vi "Accelerator Complex Process.vi"(9 "Sessions Parameters":T1={"intra_op_num_threads"=0, "inter_op_num_threads"=0, "execution_mode"=enum."ORT_SEQUENTIAL", "deterministic_compute"=FALSE, "graph_optimization_level"=1, "optimized_model_file_path"=path "", "profiling output dir"=path ""} {"graph_optimization_level" items=["ORT_DISABLE_ALL"=0, "ORT_ENABLE_ALL"=1, "ORT_ENABLE_BASIC"=2, "ORT_ENABLE_EXTENDED"=99]}, 10 "Execution Device":enum16{"CPU", "NVIDIA CUDA", "NVIDIA TensorRT"}(ring)=enum."NVIDIA CUDA", 11 "X size":i32=16384) -> (3 "Accelerator Time":dbl=1.5238084999999728)   [LabVIEW 2020]
uses:
  <vilib>/Graiphic/Accelerator/Source/ONNX/_Controls/acc_CUDA_ep_params_simplified.ctl
  <vilib>/Graiphic/Accelerator/Source/ONNX/_Controls/acc_tensorRT_ep_params_simplified.ctl
  <vilib>/Graiphic/Accelerator/Source/SubVIs/add_to_cluster_onnx_input/acc_onnx_add_1d_complexfloat_array_into_ptr_input_cluster_array_by_idx.vi
  <vilib>/Graiphic/Accelerator/Source/Model/_Methods/acc_create_onnx_model_then_init_cuda_inference_session.vi
  <vilib>/Graiphic/Accelerator/Source/Model/_Methods/acc_create_onnx_model_then_init_cpu_inference_session.vi
  <vilib>/Graiphic/Accelerator/Source/Model/_Methods/acc_create_onnx_model_then_init_tensorRT_inference_session.vi
  <vilib>/Graiphic/Accelerator/Source/SubVIs/add_to_cluster_onnx_input/acc_onnx_add_scalar_complexfloat_array_into_ptr_input_cluster_array_by_idx.vi
  <vilib>/Graiphic/Accelerator/Source/ONNX/Inference/_Methods/Simplified/acc_embedded_run_preallocated_multi_input_and_outputs_gpu_by_idx.vi
  <vilib>/Graiphic/Accelerator/Source/ONNX/Inference/_Methods/Exec_GPU/acc_embedded_copy_cuda_ptr_data_to_labview_data.vi
  <vilib>/Graiphic/Accelerator/Source/ONNX/Inference/_Methods/Simplified/acc_embedded_run_mono_output_scalar_complexfloat.vi
  <vilib>/Graiphic/Accelerator/Source/ONNX/Inference/acc_Inference.lvclass
  <vilib>/Graiphic/Accelerator/Source/Model/acc_Model.lvclass
  <vilib>/Analysis/NI_AALBase.lvlib
panel:
  in  "nb_loop":i32=6
  out "max value":csg=1.3257894e+20+1.4545643e+21i
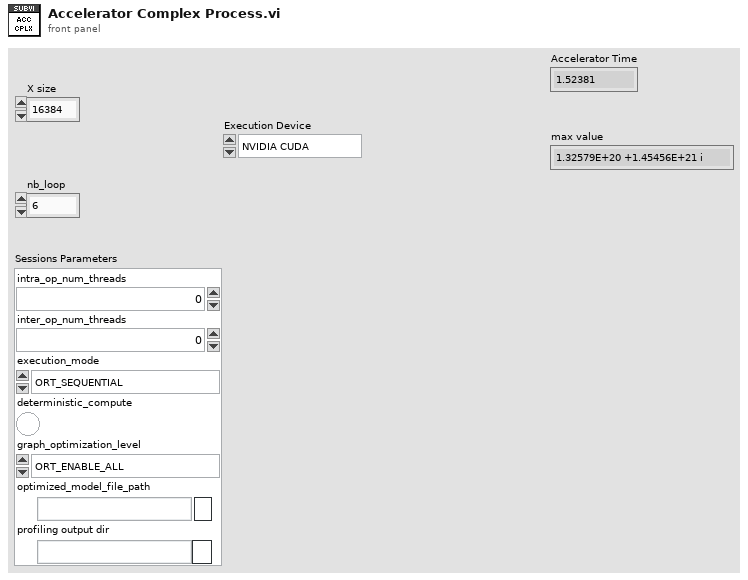
[diagram p1: front panel]
types:
  T1 = cluster{"intra_op_num_threads":i32, "inter_op_num_threads":i32, "execution_mode":enum16{"ORT_SEQUENTIAL", "ORT_PARALLEL"}, "deterministic_compute":bool, "graph_optimization_level":u16, "optimized_model_file_path":path, "profiling output dir":path}
  T2 = typedef "acc_onnx_multi_ptr_input_index_cluster.ctl" = cluster{"input_order":u32, "Inputs Info":cluster{"inputs_ptr":u64, "inputs_shapes":i64[], "inputs_ranks":i64, "inputs_types":T3}}
  T3 = typedef "acc_onnx_dtype_enum.ctl" = enum16{"UNDEFINED", "FLOAT", "UINT8", "INT8", "UINT16", "INT16", "INT32", "INT64", "STRING", "BOOL", "FLOAT16", "DOUBLE", "UINT32", "UINT64", "COMPLEX64", "COMPLEX128", "BFLOAT16", "FLOAT8E4M3FN", "FLOAT8E4M3FNUZ", "FLOAT8E5M2", "FLOAT8E5M2FNUZ", "UINT4", "INT4"}
  T4 = typedef "acc_CUDA_ep_params_simplified.ctl" = cluster{"Device & Stream":cluster{"Device Index":i32, "Use Custom Compute Stream?":bool, "Custom Compute Stream (Pointer)":u64, "Copy Using Default Stream?":bool}, "Memory Management":cluster{"GPU Memory Limit (Bytes)":u64, "Arena Extension Strategy":enum16{"kNextPowerOfTwo", "kSameAsRequested"}, "Default Memory Arena Config":u64}, "CuDNN & Kernel Optimization":cluster{"cuDNN Convolution Algorithm Search":enum16{"OrtCudnnConvAlgoSearchExhaustive", "OrtCudnnConvAlgoSearchHeuristic", "OrtCudnnConvAlgoSearchDefault"}, "Use Max Workspace for cuDNN?":bool, "Pad Conv1D Inputs to NC1D?":bool, "Fuse Convolution + Bias?":bool, "Scaled Dot-Product Attention Kernel Option":bool, "Enable Strict SkipLayerNorm Mode?":bool}, "Execution & Precision Controls":cluster{"Enable CUDA Graph Execution?":bool, "Use EP-Level Unified Stream?":bool, "Prefer NHWC Tensor Layout?":bool, "Use TensorFloat-32 (TF32)?":bool}, "Tunable Operator System":cluster{"Enable Tunable Operators?":bool, "Enable Tuning Mode for Tunable Operators?":bool, "Max Tuning Duration (ms)":i32}}
  T5 = typedef "acc_tensorRT_ep_params_simplified.ctl" = cluster{"Device And Stream":cluster{"Device Index":i32, "Use Custom Compute Stream?":bool, "Custom Compute Stream (Pointer)":u64}, "Parser & Subgraph Options":cluster{"Max Partition Attemps":i32, "Minimum Subgraph Size":i32}, "Memory & Workspace Management":cluster{"Max Workspace Memory (Bytes)":u64, "Share Memory Between Subgraphs":bool, "Auxiliary Stream Count":i32}, "Precision & Numeric Modes":cluster{"Enable FP16":bool, "Enable BF16":bool, "Enable INT8":bool, "INT8 Calibration Table Name":path, "Use Native INT8 Calibration?":bool}, "Engine Build, Cache & Paths":cluster{"Enable Engine Caching?":bool, "Engine Cache Directory":path, "Enable Engine Decryption?":bool, "Decryption Library Path":path, "Build Engines Sequentially?":bool, "Enable Timing Cache?":bool, "Timing Cache Directory":path, "Force Timing Cache Use?":bool, "Enable Detailed Logs?":bool, "Use Build Heuristics?":bool, "Enable Weight Sparsity?":bool, "Engine Optimization Level (0–5)":i32}, "Paths & Plugins":cluster{"Extra Plugin Libraries":path[], "Tactic Source Rules":string, "Enabled Preview Features":enum16{"None", "ALIASED_PLUGIN_IO_10_03"}}, "Profile Shapes":cluster{"Minimum Input Shapes":string, "Maximum Input Shapes":string, "Optimal Input Shapes":string}, "Advanced & DLA / CUDA Graph":cluster{"Enable DLA Acceleration?":bool, "DLA Core Index":i32, "Dump TensorRT Subgraphs?":bool, "Force LayerNorm in FP32?":bool, "Enable CUDA Graph Execution?":bool}}
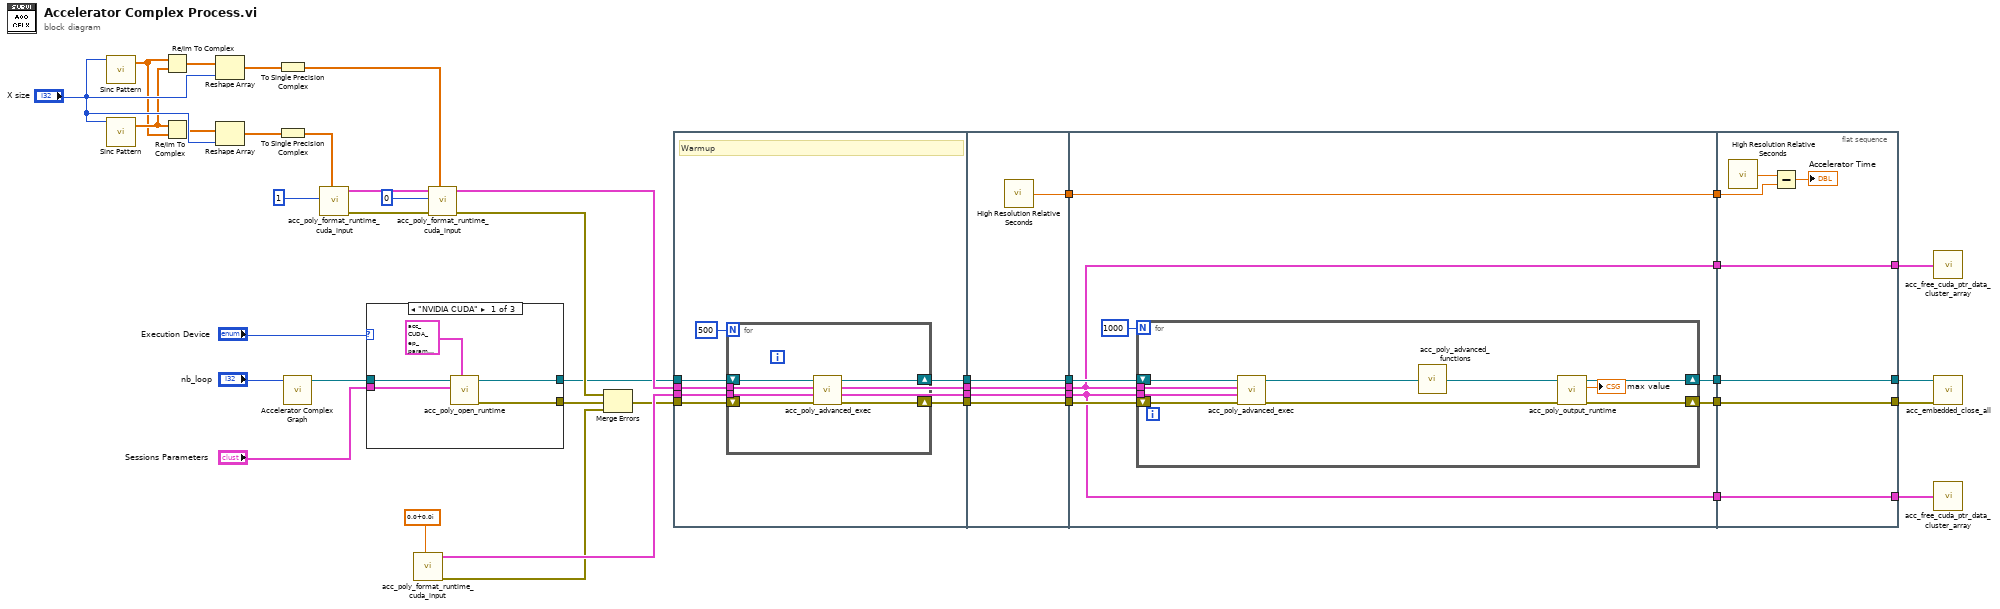
[diagram p0: block diagram]
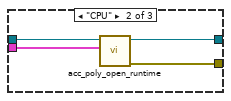
[diagram p2: hidden frame]
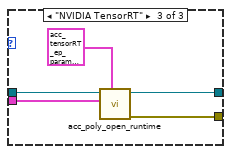
[diagram p3: hidden frame]
diagram:
  n1 = call <vilib>:"Sinc Pattern.vi"("samples"="X size") -> ("Sinc Pattern"=w11:dbl[])  [unwired: 3 in, 1 out]
  n2 = call <vilib>:"Sinc Pattern.vi"("samples"="X size") -> ("Sinc Pattern"=w12:dbl[])  [unwired: 3 in, 1 out]
  n3 = Re/Im To Complex(1:w12, 2:w11) -> (0:w13:cdb[])
  n4 = Re/Im To Complex(1:w11, 2:w12) -> (0:w10:cdb[])
  n5 = Reshape Array(w13, "X size") -> (w9:cdb[])
  n6 = Reshape Array(w10, "X size") -> (w8:cdb[])
  n7 = To Single Precision Complex(1:w9) -> (0:w6:csg[])
  n8 = To Single Precision Complex(1:w8) -> (0:w7:csg[])
  n9 = call "Accelerator Complex Graph.vi"("nb_loop"="nb_loop") -> ("Model out"=w2:refnum<class "acc_Model.lvclass">)  [unwired: 10 in]
  n10 = call-poly <vilib>:"acc_poly_format_runtime_cuda_input.vi"("1D Input Data"=w7, "input order"=1) -> ("error out"=w33:errorcluster, "Data in"=w38:T2[])  [unwired: 8 in]
  n11 = case shown="\"NVIDIA CUDA\"" "Execution Device" {
    tunnel: [w48 w52 w57] -> w5
    tunnel: [w47 w51 w56] -> w1
    tunnel: "Sessions Parameters" -> [w46 w50 w55]
    tunnel: w2 -> [w45 w49 w54]
    frame "NVIDIA CUDA" {
      n12 = call-poly <vilib>:"acc_poly_open_runtime.vi"("CUDA Parameters"=T4 {"Device & Stream"={"Device Index"=0, "Use Custom Compute Stream?"=FALSE, "Custom Compute Stream (Pointer)"=0, "Copy Using Default Stream?"=TRUE}, "Memory Management"={"GPU Memory Limit (Bytes)"=18446744073709551615, "Arena Extension Strategy"=enum."kSameAsRequested", "Default Memory Arena Config"=0}, "CuDNN & Kernel Optimization"={"cuDNN Convolution Algorithm Search"=enum."OrtCudnnConvAlgoSearchHeuristic", "Use Max Workspace for cuDNN?"=FALSE, "Pad Conv1D Inputs to NC1D?"=FALSE, "Fuse Convolution + Bias?"=FALSE, "Scaled Dot-Product Attention Kernel Option"=FALSE, "Enable Strict SkipLayerNorm Mode?"=FALSE}, "Execution & Precision Controls"={"Enable CUDA Graph Execution?"=TRUE, "Use EP-Level Unified Stream?"=FALSE, "Prefer NHWC Tensor Layout?"=FALSE, "Use TensorFloat-32 (TF32)?"=TRUE}, "Tunable Operator System"={"Enable Tunable Operators?"=FALSE, "Enable Tuning Mode for Tunable Operators?"=FALSE, "Max Tuning Duration (ms)"=0}}, "Sessions Parameters"=w46, "Model in"=w45) -> ("error out"=w47:errorcluster, "Inference out"=w48:refnum<class "acc_Inference.lvclass">)  [unwired: 7 in]
    }
    frame "CPU" {
      n13 = call-poly <vilib>:"acc_poly_open_runtime.vi"("Sessions Parameters"=w50, "Model in"=w49) -> ("error out"=w51:errorcluster, "Inference out"=w52:refnum<class "acc_Inference.lvclass">)  [unwired: 8 in]
    }
    frame "NVIDIA TensorRT" {
      n14 = call-poly <vilib>:"acc_poly_open_runtime.vi"("TRT Parameters"=T5 {"Device And Stream"={"Device Index"=0, "Use Custom Compute Stream?"=FALSE, "Custom Compute Stream (Pointer)"=0}, "Parser & Subgraph Options"={"Max Partition Attemps"=1000, "Minimum Subgraph Size"=1}, "Memory & Workspace Management"={"Max Workspace Memory (Bytes)"=0, "Share Memory Between Subgraphs"=FALSE, "Auxiliary Stream Count"=-1}, "Precision & Numeric Modes"={"Enable FP16"=FALSE, "Enable BF16"=FALSE, "Enable INT8"=FALSE, "INT8 Calibration Table Name"=path "", "Use Native INT8 Calibration?"=FALSE}, "Engine Build, Cache & Paths"={"Enable Engine Caching?"=FALSE, "Engine Cache Directory"=path "", "Enable Engine Decryption?"=FALSE, "Decryption Library Path"=path "", "Build Engines Sequentially?"=FALSE, "Enable Timing Cache?"=FALSE, "Timing Cache Directory"=path "", "Force Timing Cache Use?"=FALSE, "Enable Detailed Logs?"=FALSE, "Use Build Heuristics?"=FALSE, "Enable Weight Sparsity?"=FALSE, "Engine Optimization Level (0–5)"=3}, "Paths & Plugins"={"Extra Plugin Libraries"=[], "Tactic Source Rules"="", "Enabled Preview Features"=enum."None"}, "Profile Shapes"={"Minimum Input Shapes"="", "Maximum Input Shapes"="", "Optimal Input Shapes"=""}, "Advanced & DLA / CUDA Graph"={"Enable DLA Acceleration?"=FALSE, "DLA Core Index"=0, "Dump TensorRT Subgraphs?"=FALSE, "Force LayerNorm in FP32?"=FALSE, "Enable CUDA Graph Execution?"=FALSE}}, "Sessions Parameters"=w55, "Model in"=w54) -> ("error out"=w56:errorcluster, "Inference out"=w57:refnum<class "acc_Inference.lvclass">)  [unwired: 7 in]
    }
  }
  n15 = call-poly <vilib>:"acc_poly_format_runtime_cuda_input.vi"("Input Data"=csg 0.0+0.0i) -> ("error out"=w17:errorcluster, "Data in"=w36:T2[])  [unwired: 9 in]
  n16 = call-poly <vilib>:"acc_poly_format_runtime_cuda_input.vi"("1D Input Data"=w6, "error in"=w33, "input order"=0, "Data in"=w38) -> ("error out"=w18:errorcluster, "Data in"=w37:T2[])  [unwired: 6 in]
  n17 = Merge Errors(w18, w1, w17) -> (w31:errorcluster)
  n18 = flat-sequence {
    tunnel: w31 -> [w62]
    tunnel: w37 -> [w61]
    tunnel: w36 -> [w60]
    tunnel: w5 -> [w64]
    tunnel: [w63] -> w24
    tunnel: [w61] -> w23
    tunnel: [w60] -> w22
    tunnel: [w59] -> w21
    tunnel: [w75] -> w43
    tunnel: [w74] -> w41
    tunnel: [w73] -> w35
    tunnel: [w72] -> w34
    tunnel: [w71] -> w32
    tunnel: w24 -> [w74]
    tunnel: w23 -> [w72]
    tunnel: w22 -> [w73]
    tunnel: w21 -> [w71]
    tunnel: w43 -> [w83]
    tunnel: [w83] -> w42
    tunnel: w41 -> [w81]
    tunnel: w35 -> [w76]
    tunnel: w34 -> [w77]
    tunnel: w32 -> [w80]
    tunnel: [w79] -> w29
    tunnel: [w78] -> w28
    tunnel: [w77] -> w26
    tunnel: [w76] -> w25
    tunnel: w42 -> [w99]
    tunnel: [w97] -> w30
    tunnel: w29 -> [w97]
    tunnel: w28 -> [w96]
    tunnel: [w96] -> w27
    tunnel: [w95] -> w16
    tunnel: w26 -> [w95]
    tunnel: [w94] -> w15
    tunnel: w25 -> [w94]
    frame #0 {
      # "Warmup"
      n19 = for {
        N: 500 -> [_]
        tunnel: w61 -> [w67]
        tunnel: w60 -> [w66]
        shift-right: [w69] -> w63
        shift-left: w64 -> [w70]
        shift-right: [w65] -> w59
        shift-left: w62 -> [w68]
        n20 = call-poly <vilib>:"acc_poly_advanced_exec.vi"("error in"=w68, "Data out"=w66, "Data in"=w67, "Inference in"=w70) -> ("error out"=w65:errorcluster, "Inference out"=w69:refnum<class "acc_Inference.lvclass">)  [unwired: 6 in]
      }
    }
    frame #1 {
      n21 = call <vilib>:"High Resolution Relative Seconds.vi"() -> ("relative seconds"=w75:dbl)
    }
    frame #2 {
      n22 = for {
        N: 1000 -> [_]
        tunnel: w76 -> [w92]
        tunnel: w77 -> [w91]
        shift-right: [w87] -> w79
        shift-left: w81 -> [w93]
        shift-right: [w86] -> w78
        shift-left: w80 -> [w90]
        n23 = call-poly <vilib>:"acc_poly_advanced_exec.vi"("error in"=w90, "Data out"=w92, "Data in"=w91, "Inference in"=w93) -> ("error out"=w88:errorcluster, "Inference out"=w89:refnum<class "acc_Inference.lvclass">)  [unwired: 6 in]
        n24 = call-poly <vilib>:"acc_poly_advanced_functions.vi"("Inference in"=w89) -> ("Inference out"=w85:refnum<class "acc_Inference.lvclass">)
        n25 = call-poly <vilib>:"acc_poly_output_runtime.vi"("error in"=w88, "Inference in"=w85) -> ("error out"=w86:errorcluster, "Output Data"=→"max value":csg, "Inference out"=w87:refnum<class "acc_Inference.lvclass">)  [unwired: 7 in]
      }
    }
    frame #3 {
      n26 = call <vilib>:"High Resolution Relative Seconds.vi"() -> ("relative seconds"=w100:dbl)
      n27 = Subtract(x=w100, y=w99) -> (x-y=→"Accelerator Time":dbl)
    }
  }
  n28 = call <vilib>:"acc_free_cuda_ptr_data_cluster_array.vi"("Data in"=w16) -> ()
  n29 = call-dynamic "acc_embedded_close_all.vi"("error in"=w27, "Inference in"=w30) -> ()  [unwired: 8 in, 2 out]
  n30 = call <vilib>:"acc_free_cuda_ptr_data_cluster_array.vi"("Data in"=w15) -> ()
